vi "setInstName.vi"(8 "error in (no error)":errorcluster, 10 "Inst Name":string="lsst", 11 "OptStateEsti in":refnum<class "OptStateEsti.lvclass">) -> (0 "error out":errorcluster, 3 "OptStateEsti out":refnum<class "OptStateEsti.lvclass">)   [LabVIEW 2016, in "OptStateEsti.lvclass"]
doc: "Set the instrument name (e.g. lsst or comcam)."
uses:
  OptStateEsti.lvclass
  OptStateEsti.lvclass/OptStateEsti.ctl
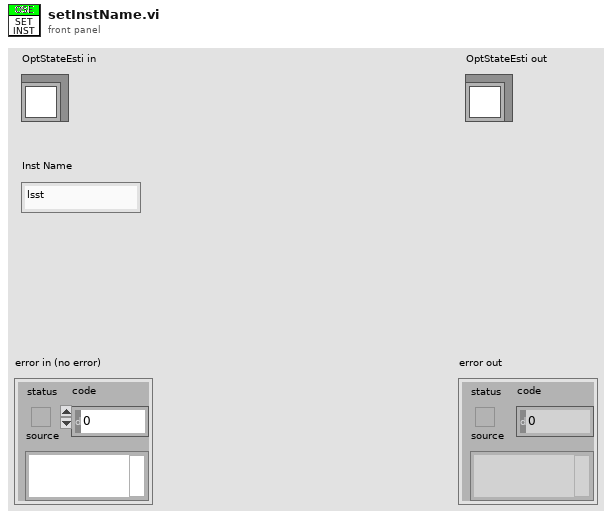
[diagram p1: front panel]
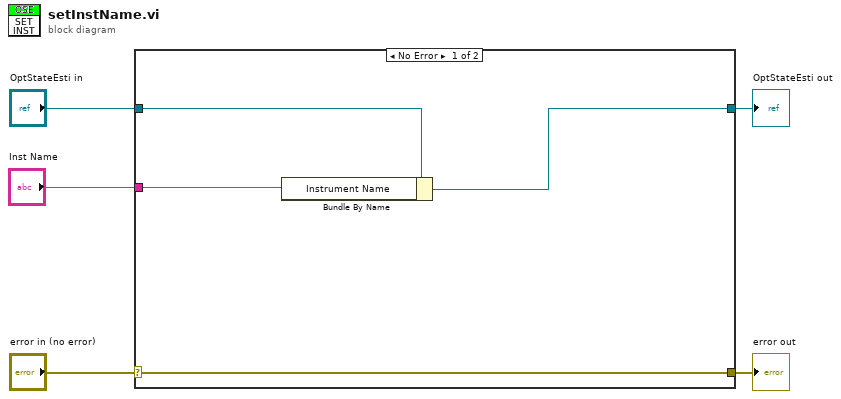
[diagram p0: block diagram]
diagram:
  n1 = case shown="No Error" "error in (no error)" {
    selector: "error in (no error)" -> [w9 w11]
    tunnel: [w9 w11] -> w4
    tunnel: [w6 w10] -> w2
    tunnel: "OptStateEsti in" -> [w7 w10]
    tunnel: "Inst Name" -> [w8 _]
    frame No Error {
      n2 = Bundle By Name(cluster=w7, "Instrument Name"=w8) -> (w6:refnum<class "OptStateEsti.lvclass">)
    }
    frame Error {
    }
  }
  "error out" <- w4
  "OptStateEsti out" <- w2
